vi "ap get io value.vi"(9 "output_value":u32, 10 "gpio_pin":u32(ring) items=["APDM_AP_GPIO_0", "APDM_AP_ANALOG_OUT_0", "APDM_AP_ANALOG_IN_0"], 11 "ap_handle":u32) -> (1 "output_value out":u32, 2 "function return":i32, 3 "ap_handle out":u32)   [LabVIEW 2019, in "apdm.lvlib"]
doc: "APDM_EXPORT int apdm_ap_get_io_value(apdm_ap_handle_t ap_handle, const apdm_ap_gpio_pin_t gpio_pin, uint32_t *output_value);"
uses:
  apdm.lvlib
  Lee Lab/CP FES Walking 2018/Code/Working/LabVIEW/apdm.dll
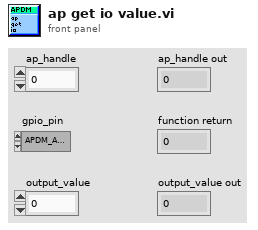
[diagram p1: front panel]
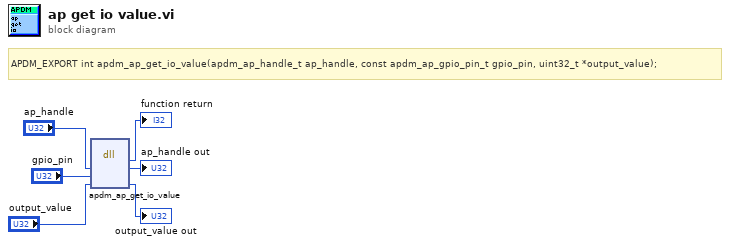
[diagram p0: block diagram]
diagram:
  # "APDM_EXPORT int apdm_ap_get_io_value(apdm_ap_handle_t ap_handle, const apdm_ap_gpio_pin_t gpio_pin, uint32_t *output_value);"
  n1 = dll-call lib="C:/Users/jfalesi/Dropbox/Lee Lab/CP FES Walking 2018/Code/Working/LabVIEW/apdm.*" fn="apdm_ap_get_io_value"("ap_handle"="ap_handle", "gpio_pin"="gpio_pin", "output_value"="output_value") -> (→"function return":i32, "ap_handle"=→"ap_handle out":u32, "output_value"=→"output_value out":u32)  [unwired: 4 in, 2 out]
